vi "LaunchObject.vi"() -> ()   [LabVIEW 2022 SP3]
uses:
  Components/ViPER.lvlibp/ViPER.lvclass
panel:
  in  "Config XML":string="<Object>\n<Name>Component_Name</Name>\n<Class>Component_Class</Class>\n</Object>"
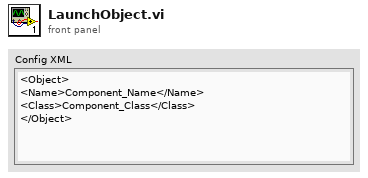
[diagram p1: front panel]
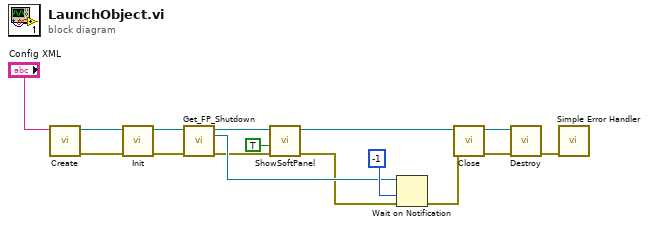
[diagram p0: block diagram]
diagram:
  n1 = call "Create.vi"("Config XML"="Config XML") -> ("error out"=w12:errorcluster, "reference out"=w13:refnum<class "ViPER.lvclass">)  [unwired: 9 in]
  n2 = call-dynamic "Init.vi"("error in (no error)"=w12, "reference in"=w13) -> ("error out"=w10:errorcluster, "reference out"=w11:refnum<class "ViPER.lvclass">)  [unwired: 8 in]
  n3 = call "Get_FP_Shutdown.vi"("ViPER_Base in"=w11, "error in (no error)"=w10) -> ("ViPER_Base out"=w8:refnum<class "ViPER.lvclass">, "SoftFP_Shutdown"=w9:refnum<notifier>, "error out"=w7:errorcluster)  [unwired: 10 in, 1 out]
  n4 = call-dynamic "ShowSoftPanel.vi"("error in (no error)"=w7, "Floating"=TRUE, "Driver in"=w8) -> ("error out"=w1:errorcluster, "Driver out"=w6:refnum<class "ViPER.lvclass">)  [unwired: 6 in, 1 out]
  n5 = Wait on Notification(notifier=w9, timeout in ms (-1)=-1, error in (no error)=w1) -> (error out=w16:errorcluster)  [unwired: 1 in, 3 out]
  n6 = call-dynamic "Close.vi"("error in (no error)"=w16, "reference in"=w6) -> ("error out"=w5:errorcluster, "reference out"=w3:refnum<class "ViPER.lvclass">)  [unwired: 8 in]
  n7 = call "Destroy.vi"("error in (no error)"=w5, "reference in"=w3) -> ("error out"=w4:errorcluster)  [unwired: 9 in]
  n8 = call <vilib>:"Simple Error Handler.vi"("error in (no error)"=w4) -> ()  [unwired: 4 in, 5 out]
